vi "Segway - Somente equilibra.vi"() -> ()   [LabVIEW 2016]
uses:
  <vilib>/NXT/Block Support/NXT_InputPort.ctl
  <vilib>/NXT/Block Support/NXT_TimerIndex.ctl
  <vilib>/NXT/Block Support/NXT_OutputPort.ctl
  <vilib>/NXT/Dual Mode Library/Waits/Wait_Num.vi
  <vilib>/NXT/Dual Mode Library/Sensors/EV3_Gyro_Reset.vi
  <vilib>/NXT/NXTIO Xnodes/NXTIONodeSubVIs/LEGOResetMotors.vi
  <vilib>/NXT/Dual Mode Library/Display/drawNumber.vi
  <vilib>/NXT/Dual Mode Library/Sensors/EV3_Gyro_Rate.vi
  <vilib>/NXT/Dual Mode Library/Motors/Rotation.vi
  <vilib>/NXT/NXTIO Xnodes/NXTIONodeSubVIs/NXTMoveMotors.vi
  <vilib>/NXT/NXTIO Xnodes/NXTIOXNode/NXTIO.xnode
  <vilib>/NXT/Subs/LVHSConnector.ctl
  <vilib>/NXT/NXTIO Xnodes/AddressXNode/NXTIOAddress.xnode
  <vilib>/NXT/LegoClasses/BrickReference/BrickReference.lvclass
panel:
  out "Impulso":dbl(graph)
  out "e":dbl
  out "Waveform Chart 2":dbl(graph) caption="Sinal para os Motores"
  out "b":dbl
  out "a":dbl
  in  "dt_program_flow":dbl
  out "dt":dbl
  out "timer_time":dbl
  out "EncSum":dbl
  out "VelAngRoda2":dbl(graph) caption="Velocidade Angular da Roda"
  out "PosAngRoda2":dbl(graph) caption="Posição Angular da Roda"
  out "PosAngCorpo2":dbl(graph) caption="Posição Angular do Corpo"
  out "VelAngCorpo2":dbl(graph) caption="Velocidade Angular do Corpo"
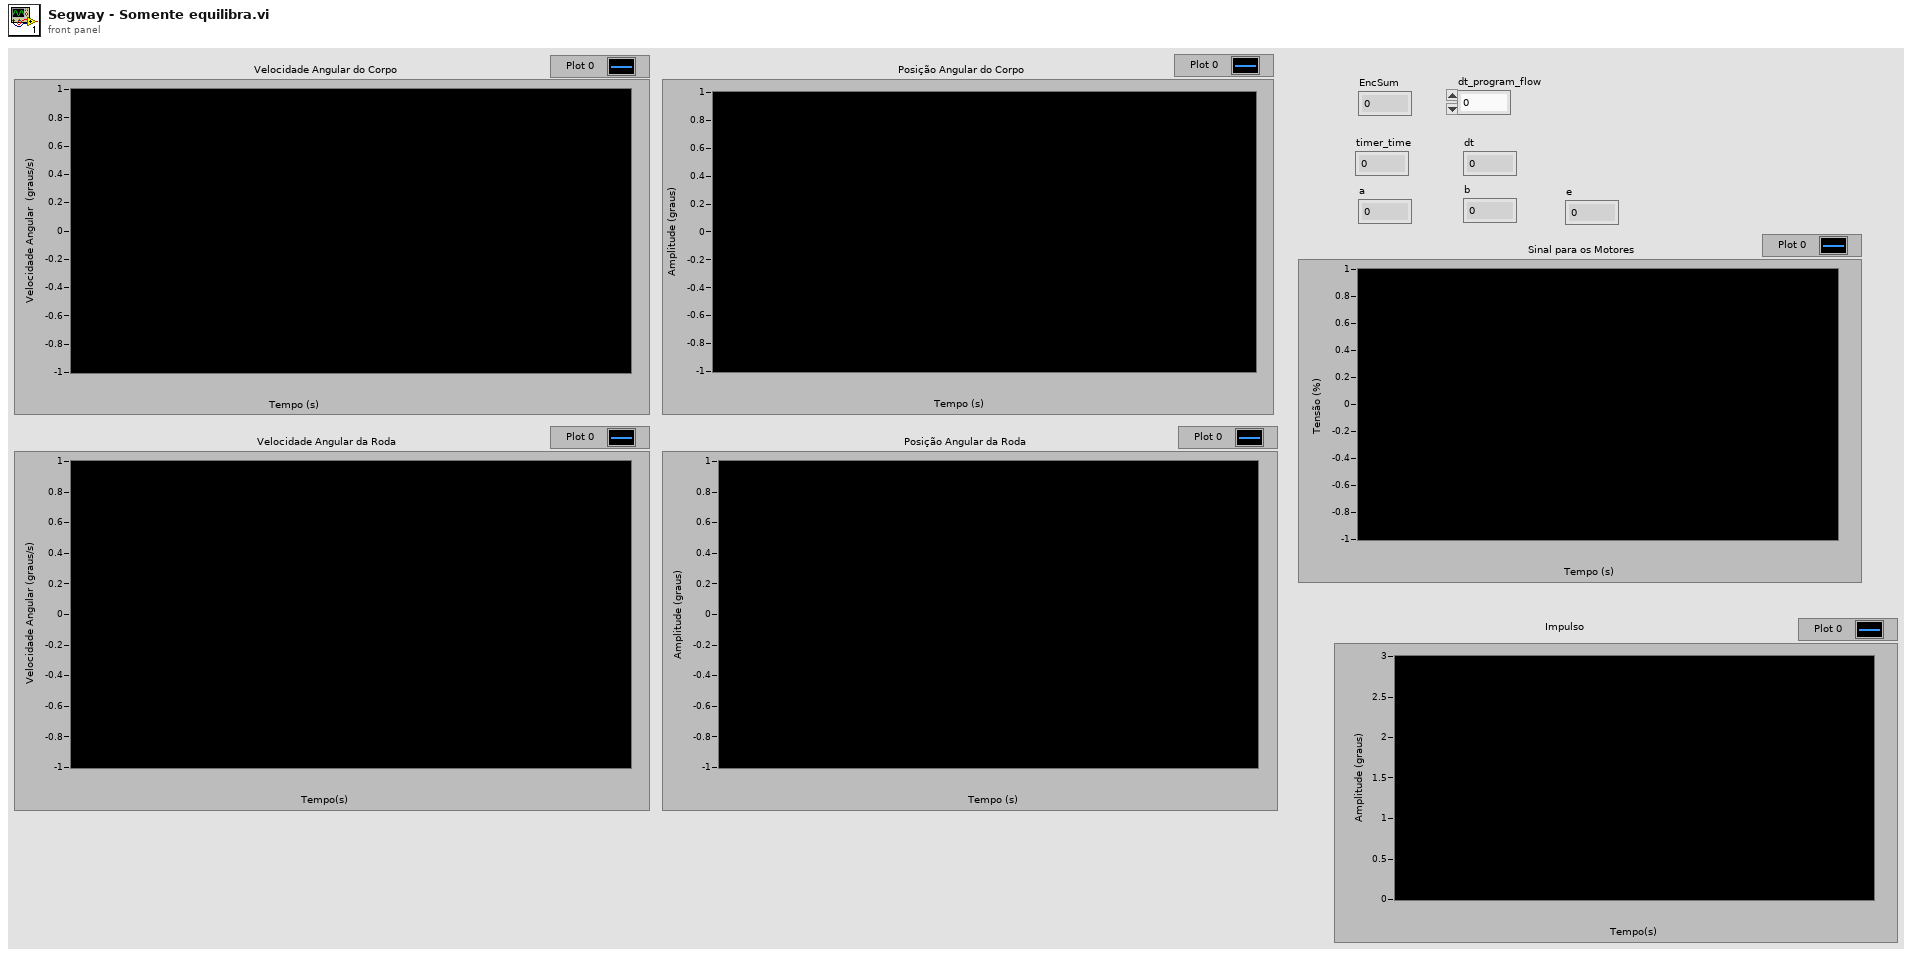
[diagram p1: front panel]
types:
  T1 = typedef "NXT_OutputPort.ctl" = u8
  T2 = typedef "NXT_TimerIndex.ctl" = u8
  T3 = typedef "NXT_InputPort.ctl" = u32
  T4 = typedef "LVHSConnector.ctl" = refnum<class "BrickReference.lvclass">
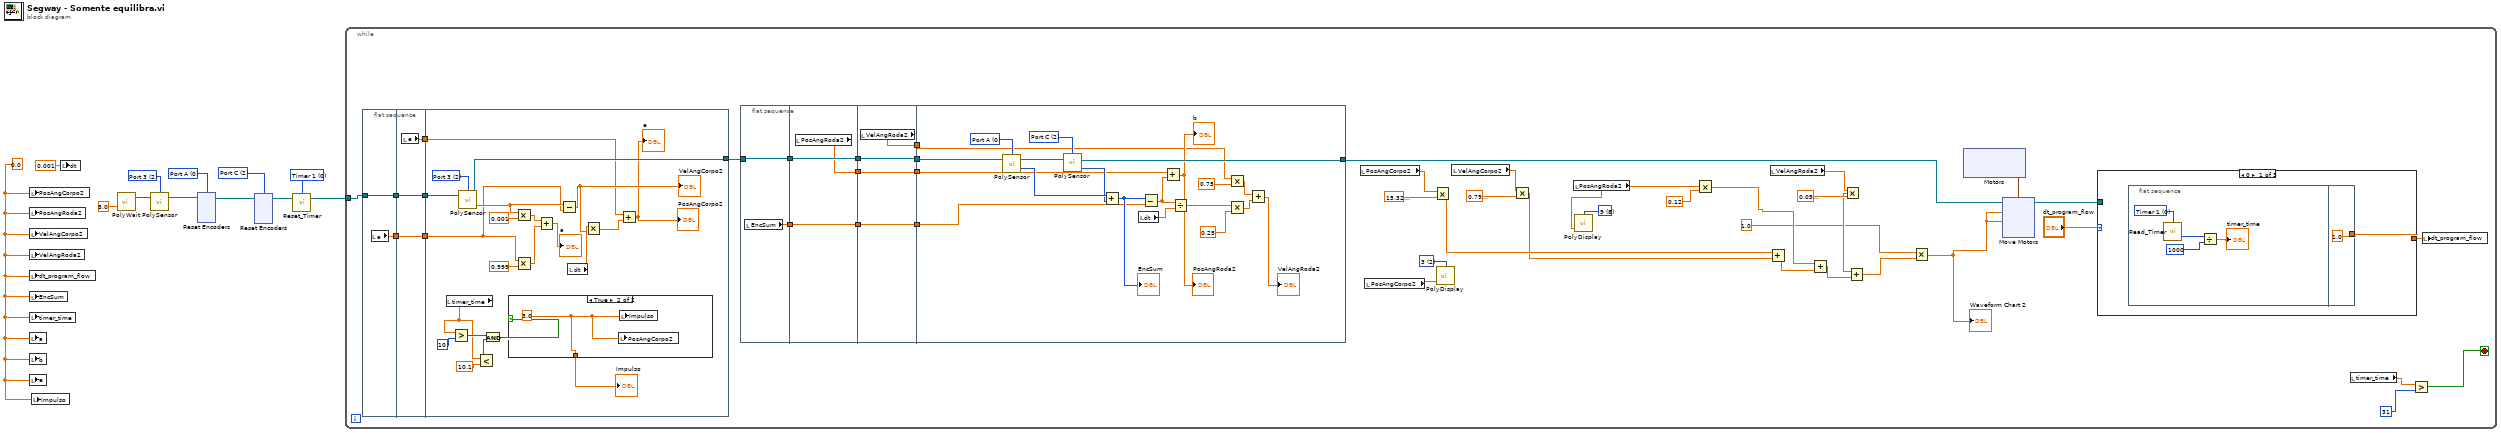
[diagram p0: block diagram]
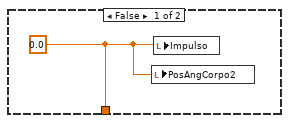
[diagram p2: hidden frame]
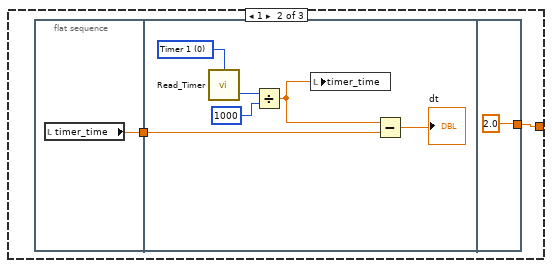
[diagram p3: hidden frame]
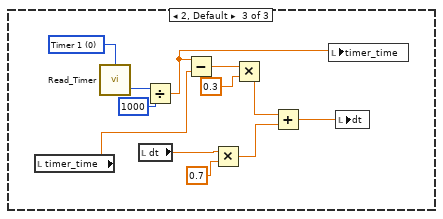
[diagram p4: hidden frame]
diagram:
  w2 = T1 0 items=["Port A", "Port B", "Port C", "Port D"] ("Port (Port A)")
  w5 = T1 2 items=["Port A", "Port B", "Port C", "Port D"] ("Port (Port A)")
  w8 = T2 0 items=["Timer 1", "Timer 2", "Timer 3"] ("Timer (Timer 1)")
  w11 = T3 2 items=["Port 1", "Port 2", "Port 3", "Port 4"] ("Port (Port 1)")
  w1 = 0.0 ("PosAngCorpo2")
  n1 = local write "PosAngCorpo2"(w1) -> ()
  n2 = local write "PosAngRoda2"(w1) -> ()
  n3 = local write "VelAngCorpo2"(w1) -> ()
  n4 = local write "VelAngRoda2"(w1) -> ()
  n5 = local write "dt_program_flow"(w1) -> ()
  n6 = local write "EncSum"(w1) -> ()
  n7 = local write "timer_time"(w1) -> ()
  n8 = local write "a"(w1) -> ()
  n9 = local write "b"(w1) -> ()
  n10 = local write "e"(w1) -> ()
  n11 = local write "Impulso"(w1) -> ()
  n12 = local write "dt"(0.001 ("dt")) -> ()
  n13 = call-poly <vilib>:"PolyWait.vi"("Time (1 sec)"=sgl 5.0) -> ("NXT/EV3"=w9:T4)  [unwired: 3 in]
  n14 = call-poly <vilib>:"PolySensor.vi"("NXT/EV3"=w9, "Port (Port 1)"=w11) -> ("NXT/EV3"=w6:T4)  [unwired: 2 in]
  n15 = xnode "Reset Encoders"("Motors"=w2, "NXT/EV3"=w6) -> ("NXT/EV3"=w4:T4)
  n16 = xnode "Reset Encoders"("Motors"=w5, "NXT/EV3"=w4) -> ("NXT/EV3"=w3:T4)
  n17 = call <vilib>:"Reset_Timer.vi"("NXT/EV3"=w3, "Timer (Timer 1)"=w8) -> ("NXT/EV3"=w7:T4)  [unwired: 2 in]
  n18 = while {
    tunnel: w7 -> [w45]
    stop <- w13 stop-if-true
    w17 = i16 8 items=["1", "2", "3", "4", "5", "6", "7", "8", "9", "10", "11", "12"] ("Line")
    w24 = i16 2 items=["1", "2", "3", "4", "5", "6", "7", "8", "9", "10", "11", "12"] ("Line")
    n19 = flat-sequence {
      tunnel: w45 -> [w87]
      tunnel: [w87] -> w39
      tunnel: [w86] -> w37
      tunnel: w39 -> [w90]
      tunnel: [w90] -> w38
      tunnel: w37 -> [w89]
      tunnel: [w89] -> w36
      tunnel: [w88] -> w35
      tunnel: [w104] -> w48
      tunnel: w38 -> [w100]
      tunnel: w36 -> [w99]
      tunnel: w35 -> [w98]
      frame #0 {
        n20 = local read "a"() -> (w86:dbl)
      }
      frame #1 {
        n21 = local read "e"() -> (w88:dbl)
      }
      frame #2 {
        w108 = T3 2 items=["Port 1", "Port 2", "Port 3", "Port 4"] ("Port (Port 1)")
        n22 = local read "timer_time"() -> (w93:dbl)
        n23 = Greater?(x=w93, y=10) -> (0:w95:bool)
        n24 = call-poly <vilib>:"PolySensor.vi"("NXT/EV3"=w100, "Port (Port 1)"=w108) -> ("Degrees/Second"=w107:sgl, "NXT/EV3"=w104:T4)  [unwired: 1 in]
        n25 = Less?(x=w93, y=10.1) -> (x < y?=w94:bool)
        n26 = And(x=w95, y=w94) -> (x .and. y?=w92:bool)
        n27 = case shown="True" w92 {
          tunnel: [w113 w114] -> w91
          frame False {
            w113 = 0.0
            n28 = local write "PosAngCorpo2"(w113) -> ()
            n29 = local write "Impulso"(w113) -> ()
          }
          frame True {
            w114 = 3.0
            n30 = local write "PosAngCorpo2"(w114) -> ()
            n31 = local write "Impulso"(w114) -> ()
          }
        }
        "Impulso" <- w91
        n32 = Multiply(x=w107, y=0.001) -> (x*y=w110:dbl)
        n33 = Multiply(x=w99, y=0.999) -> (x*y=w103:dbl)
        n34 = Add(x=w110, y=w103) -> (x+y=→"a":dbl)
        n35 = Subtract(x=w107, y=w99) -> (x-y=w105:dbl)
        "VelAngCorpo2" <- w105
        n36 = local read "dt"() -> (w106:dbl)
        n37 = Multiply(x=w106, y=w105) -> (x*y=w109:dbl)
        n38 = Add(x=w98, y=w109) -> (x+y=→"PosAngCorpo2" →"e":dbl)
      }
    }
    n39 = flat-sequence {
      tunnel: w48 -> [w58]
      tunnel: [w58] -> w34
      tunnel: [w57] -> w33
      tunnel: w34 -> [w61]
      tunnel: [w61] -> w32
      tunnel: w33 -> [w60]
      tunnel: [w60] -> w30
      tunnel: [w59] -> w27
      tunnel: w32 -> [w65]
      tunnel: [w65] -> w31
      tunnel: w30 -> [w64]
      tunnel: [w64] -> w29
      tunnel: [w63] -> w28
      tunnel: w27 -> [w62]
      tunnel: [w62] -> w26
      tunnel: w31 -> [w74]
      tunnel: [w72] -> w47
      tunnel: w29 -> [w68]
      tunnel: w28 -> [w67]
      tunnel: w26 -> [w66]
      frame #0 {
        n40 = local read "EncSum"() -> (w57:dbl)
      }
      frame #1 {
        n41 = local read "PosAngRoda2"() -> (w59:dbl)
      }
      frame #2 {
        n42 = local read "VelAngRoda2"() -> (w63:dbl)
      }
      frame #3 {
        w76 = T1 2 items=["Port A", "Port B", "Port C", "Port D"] ("Port (Port A)")
        w79 = T1 0 items=["Port A", "Port B", "Port C", "Port D"] ("Port (Port A)")
        n43 = call-poly <vilib>:"PolySensor.vi"("NXT/EV3"=w74, "Port (Port A)"=w79) -> ("Angle of Rotation"=w78:i32, "NXT/EV3"=w73:T4)  [unwired: 1 in]
        n44 = call-poly <vilib>:"PolySensor.vi"("NXT/EV3"=w73, "Port (Port A)"=w76) -> ("Angle of Rotation"=w75:i32, "NXT/EV3"=w72:T4)  [unwired: 1 in]
        n45 = Add(x=w78, y=w75) -> (x+y=w85:i32)
        "EncSum" <- w85
        n46 = local read "dt"() -> (w77:dbl)
        n47 = Subtract(x=w85, y=w68) -> (x-y=w84:dbl)
        n48 = Add(x=w66, y=w84) -> (x+y=→"PosAngRoda2" →"b":dbl)
        n49 = Divide(x=w84, y=w77) -> (x/y=w80:dbl)
        n50 = Multiply(x=w67, y=0.75) -> (x*y=w70:dbl)
        n51 = Multiply(x=w80, y=sgl 0.25) -> (x*y=w82:dbl)
        n52 = Add(x=w70, y=w82) -> (x+y=→"VelAngRoda2":dbl)
      }
    }
    n53 = local read "PosAngCorpo2"() -> (w16:dbl)
    n54 = local read "PosAngCorpo2"() -> (w25:dbl)
    n55 = Multiply(x=w16, y=sgl 15.33) -> (x*y=w44:dbl)
    n56 = call-poly <vilib>:"PolyDisplay.vi"("number"=w25, "Line"=w24) -> ()  [unwired: 2 in, 1 out]
    n57 = local read "VelAngCorpo2"() -> (w50:dbl)
    n58 = Multiply(x=w50, y=sgl 0.79) -> (x*y=w43:dbl)
    n59 = local read "PosAngRoda2"() -> (w18:dbl)
    n60 = call-poly <vilib>:"PolyDisplay.vi"("number"=w18, "Line"=w17) -> ()  [unwired: 2 in, 1 out]
    n61 = Multiply(x=w18, y=0.12) -> (x*y=w20:dbl)
    n62 = Add(x=w44, y=w43) -> (x+y=w42:dbl)
    n63 = local read "VelAngRoda2"() -> (w49:dbl)
    n64 = Add(x=w20, y=w42) -> (x+y=w41:dbl)
    n65 = Multiply(x=w49, y=sgl 0.06) -> (x*y=w40:dbl)
    n66 = Add(x=w40, y=w41) -> (x+y=w23:dbl)
    n67 = Multiply(x=1.0, y=w23) -> (x*y=w22:dbl)
    "Waveform Chart 2" <- w22
    n68 = xnode "Motors"() -> ("Motor"=w54:cluster{"Port":T1, "Port":T1})
    n69 = xnode "Move Motors"("Power/Speed 2"=w22, "Power/Speed 1"=w22, "Motors"=w54, "NXT/EV3"=w47) -> ("NXT/EV3"=w46:T4)
    n70 = case shown="0" "dt_program_flow" {
      tunnel: [w124 w130 _] -> w56
      tunnel: w46 -> [_ _ _]
      frame 0 {
        n71 = flat-sequence {
          tunnel: [1.0 ("dt_program_flow")] -> w124
          frame #0 {
            w128 = T2 0 items=["Timer 1", "Timer 2", "Timer 3"] ("Timer (Timer 1)")
            n72 = call <vilib>:"Read_Timer.vi"("Timer (Timer 1)"=w128) -> ("Value (msec)"=w125:u32)  [unwired: 2 in, 1 out]
            n73 = Divide(x=w125, y=u32 1000) -> (x/y=→"timer_time":dbl)
          }
          frame #1 {
          }
        }
      }
      frame 1 {
        n74 = flat-sequence {
          tunnel: [w132] -> w131
          tunnel: w131 -> [w138]
          tunnel: [2.0 ("dt_program_flow")] -> w130
          frame #0 {
            n75 = local read "timer_time"() -> (w132:dbl)
          }
          frame #1 {
            w136 = T2 0 items=["Timer 1", "Timer 2", "Timer 3"] ("Timer (Timer 1)")
            n76 = call <vilib>:"Read_Timer.vi"("Timer (Timer 1)"=w136) -> ("Value (msec)"=w135:u32)  [unwired: 2 in, 1 out]
            n77 = Divide(x=w135, y=u32 1000) -> (x/y=w133:dbl)
            n78 = local write "timer_time"(w133) -> ()
            n79 = Subtract(x=w133, y=w138) -> (x-y=→"dt":dbl)
          }
          frame #2 {
          }
        }
      }
      frame 2, Default {
        w143 = T2 0 items=["Timer 1", "Timer 2", "Timer 3"] ("Timer (Timer 1)")
        n80 = local read "timer_time"() -> (w140:dbl)
        n81 = call <vilib>:"Read_Timer.vi"("Timer (Timer 1)"=w143) -> ("Value (msec)"=w142:u32)  [unwired: 2 in, 1 out]
        n82 = local read "dt"() -> (w145:dbl)
        n83 = Divide(x=w142, y=u32 1000) -> (x/y=w150:dbl)
        n84 = Subtract(x=w150, y=w140) -> (x-y=w149:dbl)
        n85 = Multiply(x=w145, y=0.7) -> (x*y=w144:dbl)
        n86 = Multiply(x=w149, y=0.3) -> (x*y=w147:dbl)
        n87 = Add(x=w147, y=w144) -> (x+y=w151:dbl)
        n88 = local write "timer_time"(w150) -> ()
        n89 = local write "dt"(w151) -> ()
      }
    }
    n90 = local read "timer_time"() -> (w15:dbl)
    n91 = Greater?(x=w15, y=31) -> (0:w13:bool)
    n92 = local write "dt_program_flow"(w56) -> ()
  }
